vi "Get Current Shift ver3.vi"(10 "Base File Path":path) -> (0 "Current Shift Number":u32, 1 "Shift":string, 3 "refnum out":T1)   [LabVIEW 2018]
uses:
  <vilib>/Utility/config.llb/Config Data RefNum.ctl
  <vilib>/Utility/config.llb/Read Key (String).vi
  <vilib>/Utility/config.llb/NI_LVConfig.lvlib
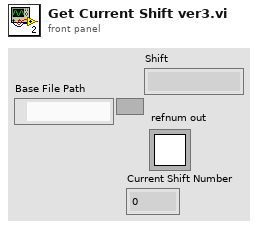
[diagram p1: front panel]
types:
  T1 = typedef "NI_LVConfig.lvlib/Config Data RefNum.ctl" = refnum<k1>
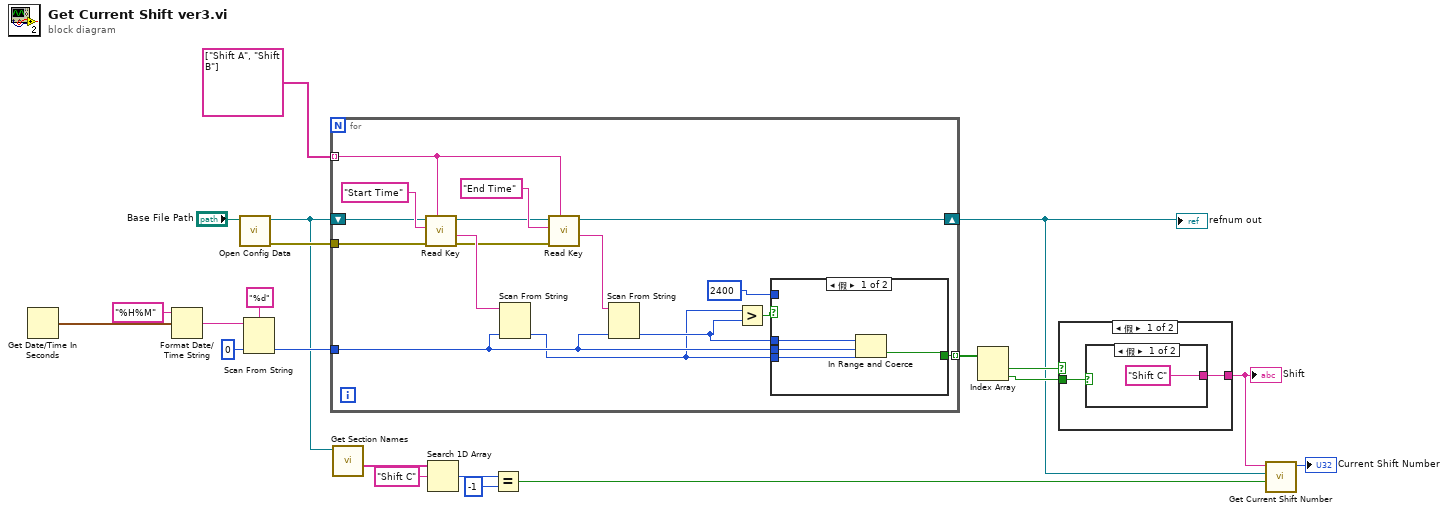
[diagram p0: block diagram]
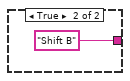
[diagram p2: hidden frame]
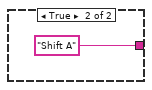
[diagram p3: hidden frame]
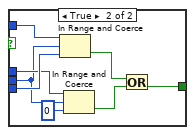
[diagram p4: hidden frame]
diagram:
  n1 = Get Date/Time In Seconds() -> (seconds since 1Jan1904=w10:timestamp)
  n2 = Format Date/Time String(time format string (%c)="%H%M", seconds (now)=w10) -> (date/time string=w18:string)  [unwired: 1 in]
  n3 = call <vilib>:"Open Config Data.vi"("configuration file path"="Base File Path") -> ("error out"=w21:errorcluster, "refnum"=w9:T1)  [unwired: 8 in, 1 out]
  n4 = Scan From String(format string="%d", input string=w18, default 1=u32 0 ("default value 1")) -> (output 1=w15:u32)  [unwired: 2 in, 3 out]
  n5 = for {
    tunnel: string[] ["Shift A", "Shift B"] -> [w34] mode=indexing
    tunnel: w21 -> [w31]
    tunnel: [w25] -> w13 mode=indexing
    tunnel: w15 -> [w23]
    shift-right: [w28] -> w1
    shift-left: w9 -> [w29]
    n6 = call-poly <vilib>:"Read Key.vi"("section"=w34, "error in (no error)"=w31, "key"="Start Time", "refnum"=w29) -> ("error out"=w33:errorcluster, "value"=w36:string, "refnum out"=w32:T1)  [unwired: 4 in, 1 out]
    n7 = Scan From String(input string=w36, default 1=w23) -> (output 1=w22:u32)  [unwired: 3 in, 3 out]
    n8 = call-poly <vilib>:"Read Key.vi"("section"=w34, "error in (no error)"=w33, "key"="End Time", "refnum"=w32) -> ("value"=w37:string, "refnum out"=w28:T1)  [unwired: 4 in, 2 out]
    n9 = Scan From String(input string=w37, default 1=w23) -> (output 1=w24:u32)  [unwired: 3 in, 3 out]
    n10 = Greater?(x=w22, y=w24) -> (0:w27:bool)
    n11 = case shown="假" w27 {
      tunnel: [w38 w44] -> w25
      tunnel: w23 -> [w40 w46]
      tunnel: w22 -> [w39 w49]
      tunnel: w24 -> [w41 w47]
      tunnel: u32 2400 ("y") -> [_ w48]
      frame False {
        n12 = In Range and Coerce(upper limit=w41, x=w40, lower limit=w39) -> (In Range?=w38:bool)  [unwired: 1 out]
      }
      frame True {
        n13 = In Range and Coerce(upper limit=w48, x=w46, lower limit=w49) -> (In Range?=w43:bool)  [unwired: 1 out]
        n14 = In Range and Coerce(upper limit=w47, x=w46, lower limit=u32 0) -> (In Range?=w42:bool)  [unwired: 1 out]
        n15 = Or(x=w43, y=w42) -> (x .or. y?=w44:bool)
      }
    }
  }
  "refnum out" <- w1
  n16 = call <vilib>:"Get Section Names.vi"("refnum"=w9) -> ("section names"=w8:string[])  [unwired: 8 in, 2 out]
  n17 = Search 1D Array(1D array=w8, element="Shift C") -> (index of element=w6:i32)  [unwired: 1 in]
  n18 = Equal?(x=w6, y=-1) -> (x = y?=w3:bool)
  n19 = Index Array(array=w13) -> (element #1=w12:bool, element #2=w11:bool)  [unwired: 2 in]
  n20 = case shown="假" w12 {
    tunnel: [w50 "Shift A" ("section")] -> w4
    tunnel: w11 -> [w51 _]
    frame False {
      n21 = case shown="假" w51 {
        tunnel: ["Shift C" ("section") "Shift B" ("section")] -> w50
        frame False {
        }
        frame True {
        }
      }
    }
    frame True {
    }
  }
  "Shift" <- w4
  n22 = call "Get Current Shift Number.vi"("Two Shift Pattern"=w3, "refnum in"=w1, "Shift"=w4) -> ("Numeric"=→"Current Shift Number":u32)  [unwired: 8 in]
